vi "KIT-QVA-Content.vi"() -> (0 "CS++Classes & Messages":T1(array[cluster]))   [LabVIEW 2014]
doc: "Place actor and class constants that should be included included in an application on the blockdiagramm."
uses:
  <vilib>/ActorFramework/Message/Message.lvclass
  KIT-QVA/KIT-QVA.lvclass
  KIT-QVG/KIT-QVG.lvclass
  CSPP_Core/Actors/CS++BaseActor/CS++BaseActor.lvclass
panel:
  # "Place actor and class constants on the blockdiagramm."
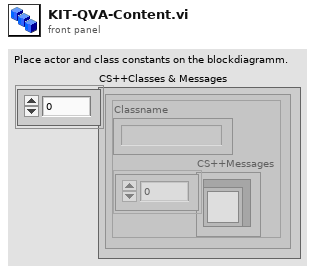
[diagram p1: front panel]
types:
  T1 = cluster{"Classname":string, "CS++Messages":refnum<class "Message.lvclass">[]}[]
  T2 = cluster{"class name":string, "CS++Messages":refnum<class "Message.lvclass">[]}
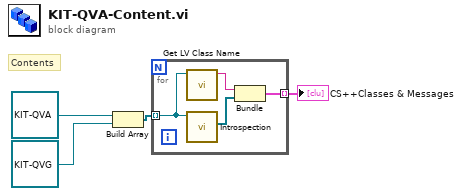
[diagram p0: block diagram]
diagram:
  # "Contents"
  n1 = Build Array(refnum<class "KIT-QVA.lvclass"> refnum ("KIT-QVA.lvlib:KIT-QVA.lvclass"), refnum<class "KIT-QVG.lvclass"> refnum ("KIT-QVG.lvlib:KIT-QVG.lvclass")) -> (w3:refnum<class "CS++BaseActor.lvclass">[])
  n2 = for {
    tunnel: w3 -> [w8] mode=indexing
    tunnel: [w5] -> w4 mode=indexing
    n3 = call <vilib>:"Get LV Class Name.vi"("object"=w8) -> ("class name"=w7:string)  [unwired: 9 in, 1 out]
    n4 = call "Introspection.vi"("CS++BaseActor in"=w8) -> ("CS++Messages"=w6:refnum<class "Message.lvclass">[])  [unwired: 8 in, 2 out]
    n5 = Bundle("class name"=w7, "CS++Messages"=w6) -> (w5:T2)  [unwired: 1 in]
  }
  "CS++Classes & Messages" <- w4
